vi "Fuente.vi"(1 "DC OK":string) -> (0 "String":string)   [LabVIEW 2015]
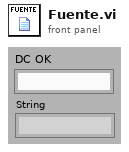
[diagram p1: front panel]
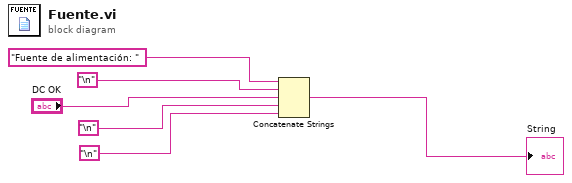
[diagram p0: block diagram]
diagram:
  n1 = Concatenate Strings("Fuente de alimentación: ", "\n", "DC OK", "\n", "\n") -> (→"String":string)
